vi "_039.vi"() -> ()   [LabVIEW 2024]
panel:
  in  "stop":bool
  out "Boolean":bool
  out "Tank":dbl(slide) scale=0.0..100.0
  in  "Boolean 2":bool
  # "Level of water tank was monitered by LED :"
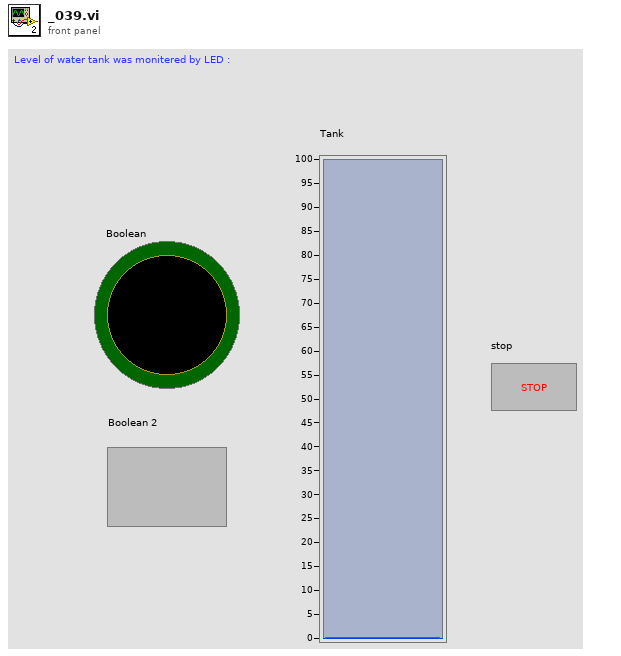
[diagram p1: front panel]
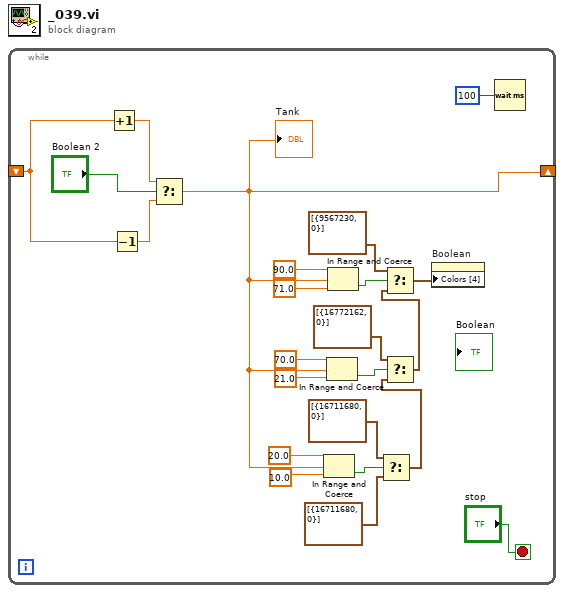
[diagram p0: block diagram]
diagram:
  n1 = while {
    shift-right: [w20] -> _
    shift-left: _ -> [w1]
    stop <- "stop" stop-if-true
    n2 = Increment(x=w1) -> (x+1=w21:dbl)
    n3 = Decrement(x=w1) -> (x-1=w22:dbl)
    n4 = Select(t=w21, s="Boolean 2", f=w22) -> (s? t:f=w20:dbl)
    "Tank" <- w20
    n5 = In Range and Coerce(upper limit=20.0, x=w20, lower limit=10.0 ("upper limit")) -> (In Range?=w11:bool)  [unwired: 1 out]
    n6 = In Range and Coerce(upper limit=70.0, x=w20, lower limit=21.0 ("upper limit")) -> (In Range?=w12:bool)  [unwired: 1 out]
    n7 = In Range and Coerce(upper limit=90.0, x=w20, lower limit=71.0 ("upper limit")) -> (In Range?=w13:bool)  [unwired: 1 out]
    n8 = Select(t=cluster{u32, u32}[] [{16711680, 0}] ("Colors [4]"), s=w11, f=cluster{u32, u32}[] [{16711680, 0}] ("Colors [4]")) -> (s? t:f=w6:cluster{u32, u32}[])
    n9 = Select(t=cluster{u32, u32}[] [{16772162, 0}] ("Colors [4]"), s=w12, f=w6) -> (s? t:f=w5:cluster{u32, u32}[])
    n10 = Select(t=cluster{u32, u32}[] [{9567230, 0}] ("Colors [4]"), s=w13, f=w5) -> (s? t:f=w4:cluster{u32, u32}[])
    n11 = property on="Boolean" class="Bool (strict)"("Colors [4]"=w4) -> ()  [unwired: 2 in, 2 out]
    n12 = Wait (ms)(milliseconds to wait=u32 100 ("millisecond timer value")) -> ()  [unwired: 1 out]
  }
